vi "Process Job.vi"(8 "error in (no error)":errorcluster, 10 "Task":refnum<class>, 11 "Mock Worker In":refnum<class "Mock Worker.lvclass">) -> (0 "error out":errorcluster, 3 "Mock Worker Out":refnum<class "Mock Worker.lvclass">)   [LabVIEW 2020, in "Mock Worker.lvclass"]
uses:
  Mock Worker.lvclass
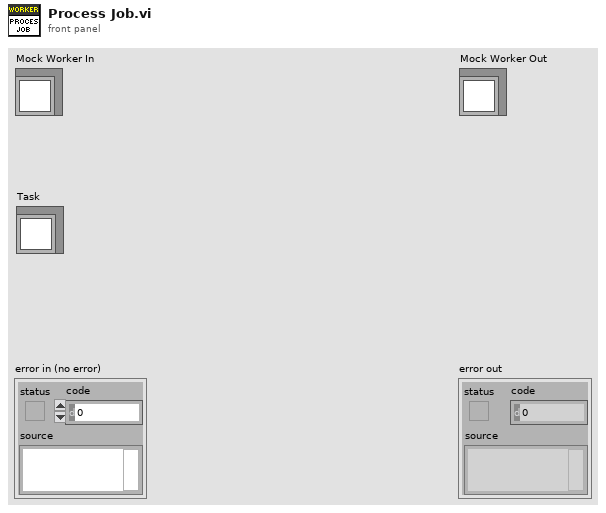
[diagram p1: front panel]
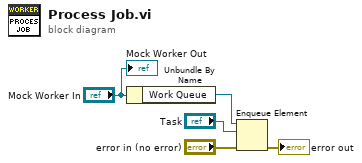
[diagram p0: block diagram]
diagram:
  n1 = Unbundle By Name("Mock Worker In") -> ("Work Queue"=w4:refnum<queue>)
  n2 = Enqueue Element(queue=w4, element="Task", error in (no error)="error in (no error)") -> (error out=→"error out":errorcluster)  [unwired: 1 in, 2 out]
  "Mock Worker Out" <- "Mock Worker In"
